vi "Write TableData.vi"(8 "error in (no error)":errorcluster, 10 "TableData":string[][](array[string]), 11 "Instruments in":refnum<class "Instruments.lvclass">) -> (0 "error out":errorcluster, 3 "Instruments out":refnum<class "Instruments.lvclass">)   [LabVIEW 2023, in "Instruments.lvlib" / "Instruments.lvclass"]
uses:
  Library/Instruments.lvclass
  Library/Instruments.lvclass/Instruments.ctl
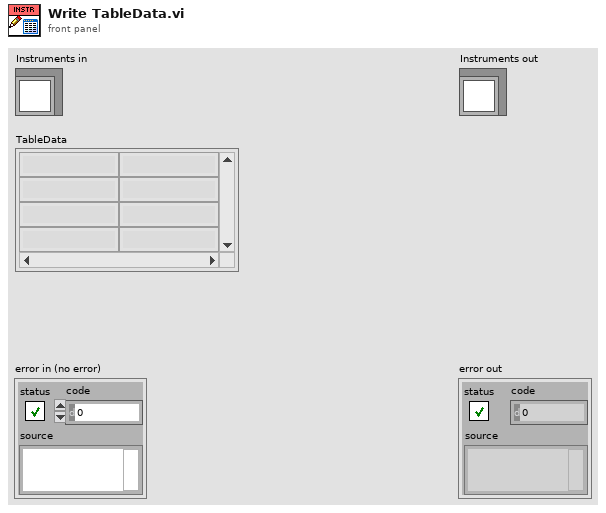
[diagram p1: front panel]
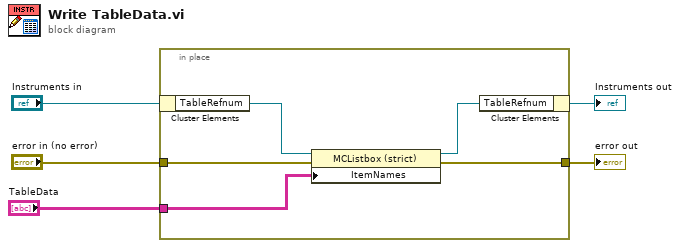
[diagram p0: block diagram]
diagram:
  n1 = in-place {
    in-place-border: "error in (no error)" -> [w8]
    in-place-border: [w7] -> w2
    in-place-border: "TableData" -> [w6]
    n2 = in-place-cluster #1("Instruments in") -> ("TableRefnum"=w10:refnum<vi>)
    n3 = property class="MCListbox (strict)"(reference=w10, error in=w8, "ItemNames"=w6) -> (reference out=w9:refnum<vi>, error out=w7:errorcluster)
    n4 = in-place-cluster #1("TableRefnum"=w9) -> (→"Instruments out":refnum<class "Instruments.lvclass">)
  }
  "error out" <- w2
